vi "AODO-Write (DO).vi"(0 "Task In":refnum<k21>, 7 "DO Waveforms":bool[][](array[boolean]), 11 "error in (no error)":errorcluster) -> (4 "Task Out":refnum<k21>, 15 "error out":errorcluster)   [LabVIEW 2020]
uses:
  <vilib>/DAQmx/write.llb/DAQmx Write (Digital Wfm 1Chan NSamp).vi
  <vilib>/Waveform/DWDTOps.llb/DWDT Boolean Array to Digital.vi
  <vilib>/Waveform/DWDTOps.llb/DWDT Uncompress Digital.vi
  <vilib>/DAQmx/miscellaneous.llb/DAQmx Fill In Error Info.vi
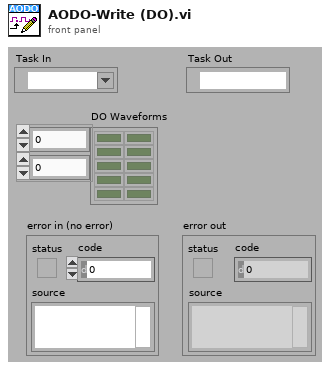
[diagram p1: front panel]
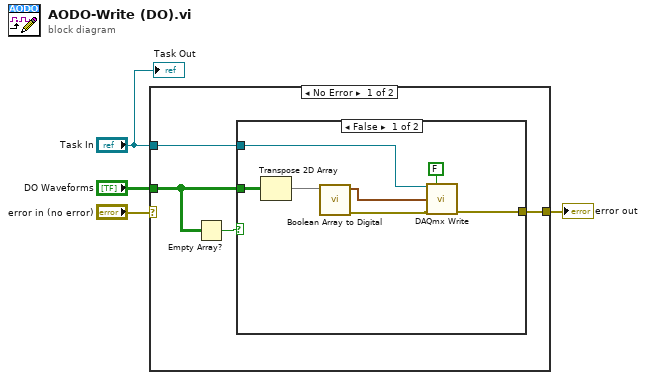
[diagram p0: block diagram]
diagram:
  n1 = case shown="No Error" "error in (no error)" {
    selector: "error in (no error)" -> [_ w16]
    tunnel: [w8 w16] -> w4
    tunnel: "DO Waveforms" -> [w6 _]
    tunnel: "Task In" -> [w5 _]
    frame No Error {
      n2 = Empty Array?(array=w6) -> (empty?=w7:bool)
      n3 = case shown="False" w7 {
        tunnel: w5 -> [w9 _]
        tunnel: [w11 _] -> w8
        tunnel: w6 -> [w10 _]
        frame False {
          n4 = Transpose 2D Array(2D array=w10) -> (transposed array=w12:bool[][])
          n5 = call-poly <vilib>:"Boolean Array to Digital.vi"("boolean array"=w12) -> ("error out"=w15:errorcluster, "digital waveform"=w13:digitalwaveform)  [unwired: 9 in]
          n6 = call-poly <vilib>:"DAQmx Write.vi"("task/channels in"=w9, "auto start"=FALSE, "data"=w13, "error in"=w15) -> ("error out"=w11:errorcluster)  [unwired: 9 in, 2 out]
        }
        frame True {
        }
      }
    }
    frame Error {
    }
  }
  "error out" <- w4
  "Task Out" <- "Task In"
